vi "To Pythonic - Integer.vi"(4 "Integer":i64) -> (1 "Pythonic Value":string)   [LabVIEW 2012, in "OPI.lvclass"]
doc: "Convert LabVIEW data into valid pythonic representation."
uses:
  OPI.lvclass
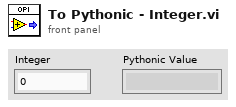
[diagram p1: front panel]
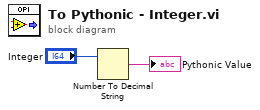
[diagram p0: block diagram]
diagram:
  n1 = Number To Decimal String(number="Integer") -> (decimal integer string=→"Pythonic Value":string)  [unwired: 1 in]
